vi "test_OpenClose (Multi Sessions) 2.vi"() -> ()   [LabVIEW 2020]
uses:
  <instrlib>/AIM GmbH/_AIM 664/AIM664LV.lvlib
  <instrlib>/AIM GmbH/_AIM 664/bsp/Fdx Create Session (Tx-Generic).vi
panel:
  in  "board 2":u32
  in  "port 2":u32
  in  "port":u32
  in  "board":u32
  out "executed":i32
  in  "Iterations":i32=1
  in  "idle before iterations mS":u32=1000
  out "error out 2":errorcluster caption="error out"
  out "error out":errorcluster
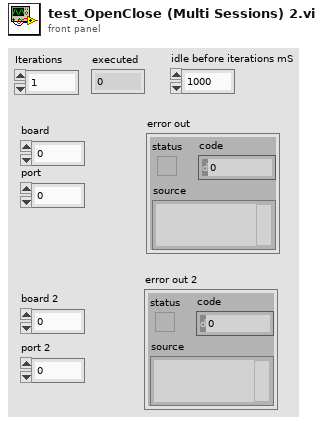
[diagram p1: front panel]
types:
  T1 = cluster{"ReceiveMode":u32, "DefaultPayloadMode":u32, "DefaultCronoMode":u32, "GlbMonBufferSizeIn":u32, "RerosDefaultOutputPortmap":u32}
  T2 = cluster{"ResourceID":u32, "ResourceType":u32, "ResourceInfo":string, "StructId":u32}
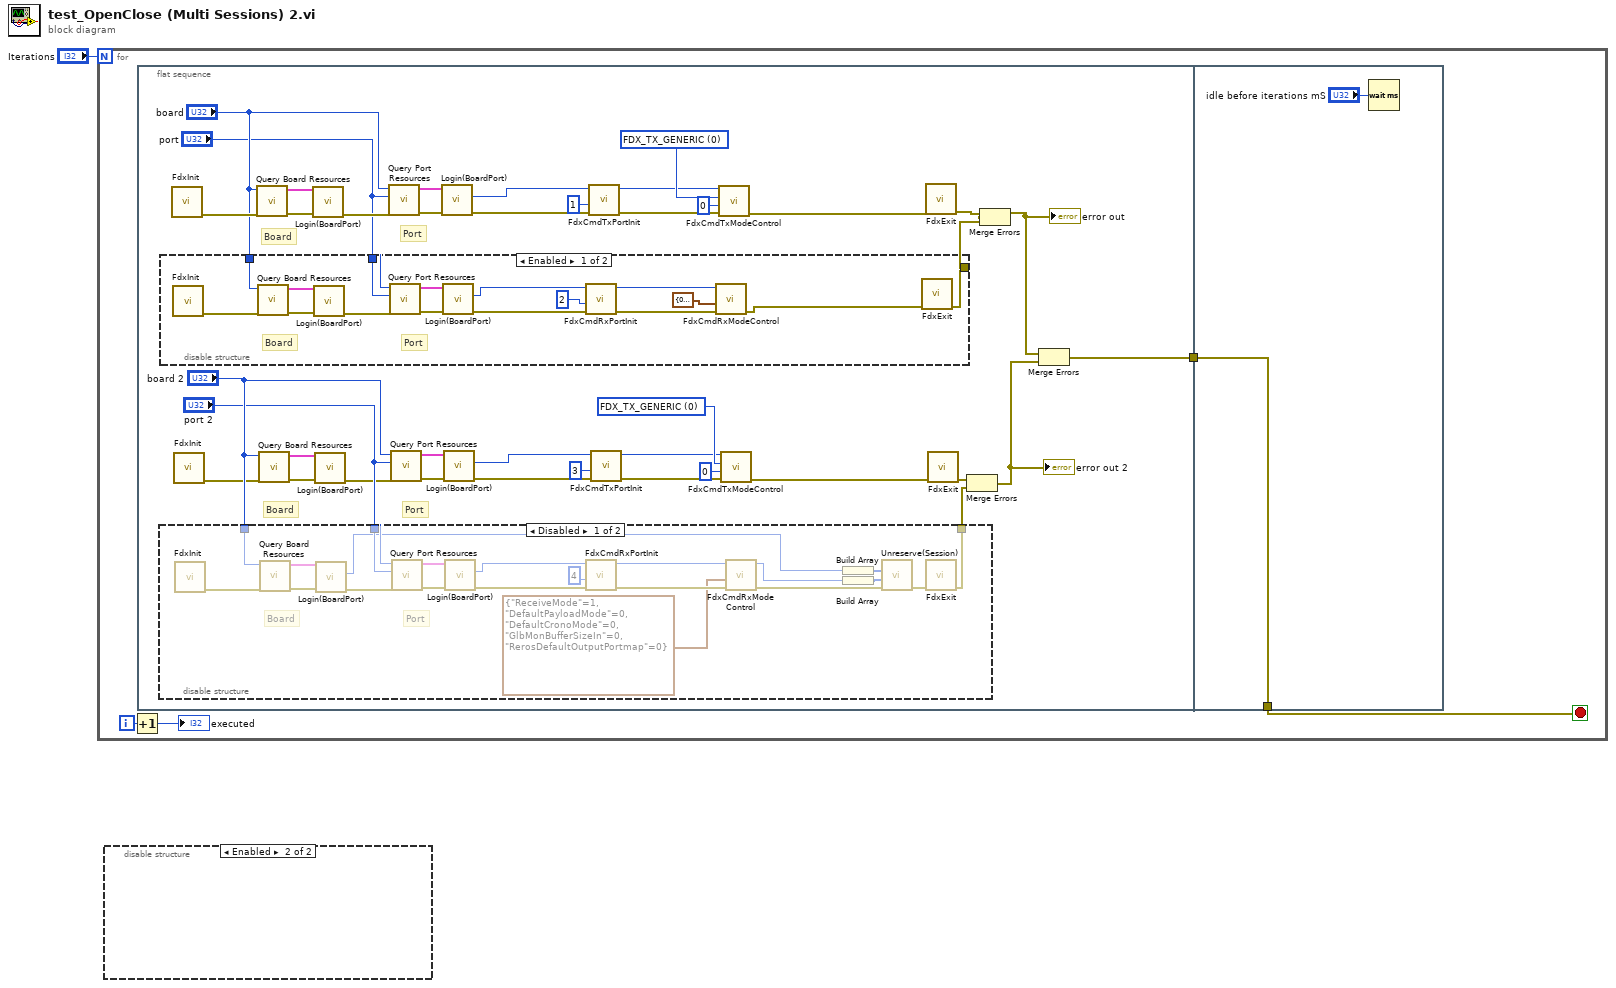
[diagram p0: block diagram]
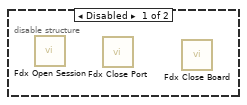
[diagram p4: hidden frame]
diagram:
  n1 = for {
    N: "Iterations" -> [_]
    i -> [w3]
    stop <- w5 stop-if-true
    n2 = Increment(x=w3) -> (x+1=→"executed":i32)
    n3 = flat-sequence {
      tunnel: [w44] -> w4
      tunnel: [w82] -> w5
      tunnel: w4 -> [w82]
      frame #0 {
        w28 = u32 0 items=["FDX_TX_GENERIC", "FDX_TX_REPLAY", "FDX_TX_INDIVIDUAL"] ("TransmitMode")
        w36 = u32 0 items=["FDX_TX_GENERIC", "FDX_TX_REPLAY", "FDX_TX_INDIVIDUAL"] ("TransmitMode")
        # "Port"
        # "Board"
        # "Port"
        # "Board"
        n4 = disable-structure shown="Disabled" {
          disable-tunnel: "board 2" -> [w75 _]
          disable-tunnel: "port 2" -> [w74 _]
          disable-tunnel: [w64 _] -> w22
          frame Disabled {
            # "Port"
            # "Board"
            n5 = call <instrlib>:"FdxInit.vi"() -> ("error out"=w81:errorcluster)  [unwired: 10 in, 1 out]
            n6 = call <instrlib>:"Query Board Resources.vi"("error in (no error)"=w81, "board"=w75) -> ("error out"=w80:errorcluster, "board resource"=w79:T2)  [unwired: 7 in, 1 out]
            n7 = call <instrlib>:"Login(BoardPort).vi"("error in (no error)"=w80, "resource in"=w79) -> ("error out"=w78:errorcluster, "Handle"=w70:u32)  [unwired: 7 in, 1 out]
            n8 = call <instrlib>:"Query Port Resources.vi"("error in (no error)"=w78, "port"=w74, "board"=w75) -> ("error out"=w77:errorcluster, "port resource"=w76:T2)  [unwired: 6 in, 1 out]
            n9 = call <instrlib>:"Login(BoardPort).vi"("error in (no error)"=w77, "resource in"=w76) -> ("error out"=w69:errorcluster, "Handle"=w62:u32)  [unwired: 7 in, 1 out]
            n10 = call <instrlib>:"FdxCmdRxPortInit.vi"("error in"=w69, "PortMap"=u32 4, "InstrumentHandle_port in"=w62) -> ("error out"=w68:errorcluster, "InstrumentHandle_port out"=w63:u32)  [unwired: 6 in, 1 out]
            n11 = call <instrlib>:"FdxCmdRxModeControl.vi"("error in"=w68, "RxModeControlIn"=T1 {"ReceiveMode"=1, "DefaultPayloadMode"=0, "DefaultCronoMode"=0, "GlbMonBufferSizeIn"=0, "RerosDefaultOutputPortmap"=0}, "InstrumentHandle_port in"=w63) -> ("error out"=w67:errorcluster, "InstrumentHandle_port out"=w66:u32)  [unwired: 6 in, 1 out]
            n12 = Build Array(w70) -> (w71:u32[])
            n13 = Build Array(w66) -> (w72:u32[])
            n14 = call <instrlib>:"Unreserve(Session).vi"("error in (no error)"=w67, "InstrumentHandle_port in"=w72, "InstrumentHandle_board in"=w71) -> ("error out"=w73:errorcluster)  [unwired: 8 in]
            n15 = call <instrlib>:"FdxExit.vi"("error in"=w73) -> ("error out"=w64:errorcluster)  [unwired: 10 in]
          }
          frame Enabled {
          }
        }
        n16 = disable-structure shown="Enabled" {
          disable-tunnel: [w52 _] -> w23
          disable-tunnel: "board" -> [w51 _]
          disable-tunnel: "port" -> [w50 _]
          frame Enabled {
            # "Port"
            # "Board"
            n17 = call <instrlib>:"FdxInit.vi"() -> ("error out"=w55:errorcluster)  [unwired: 10 in, 1 out]
            n18 = call <instrlib>:"Query Board Resources.vi"("error in (no error)"=w55, "board"=w51) -> ("error out"=w56:errorcluster, "board resource"=w57:T2)  [unwired: 7 in, 1 out]
            n19 = call <instrlib>:"Login(BoardPort).vi"("error in (no error)"=w56, "resource in"=w57) -> ("error out"=w58:errorcluster)  [unwired: 7 in, 2 out]
            n20 = call <instrlib>:"Query Port Resources.vi"("error in (no error)"=w58, "port"=w50, "board"=w51) -> ("error out"=w59:errorcluster, "port resource"=w60:T2)  [unwired: 6 in, 1 out]
            n21 = call <instrlib>:"Login(BoardPort).vi"("error in (no error)"=w59, "resource in"=w60) -> ("error out"=w54:errorcluster, "Handle"=w49:u32)  [unwired: 7 in, 1 out]
            n22 = call <instrlib>:"FdxCmdRxPortInit.vi"("error in"=w54, "PortMap"=u32 2, "InstrumentHandle_port in"=w49) -> ("error out"=w53:errorcluster, "InstrumentHandle_port out"=w47:u32)  [unwired: 6 in, 1 out]
            n23 = call <instrlib>:"FdxCmdRxModeControl.vi"("error in"=w53, "RxModeControlIn"=T1 {"ReceiveMode"=0, "DefaultPayloadMode"=0, "DefaultCronoMode"=0, "GlbMonBufferSizeIn"=0, "RerosDefaultOutputPortmap"=0}, "InstrumentHandle_port in"=w47) -> ("error out"=w46:errorcluster)  [unwired: 6 in, 2 out]
            n24 = call <instrlib>:"FdxExit.vi"("error in"=w46) -> ("error out"=w52:errorcluster)  [unwired: 10 in]
          }
          frame Disabled {
          }
        }
        n25 = call <instrlib>:"FdxInit.vi"() -> ("error out"=w43:errorcluster)  [unwired: 10 in, 1 out]
        n26 = call <instrlib>:"FdxInit.vi"() -> ("error out"=w7:errorcluster)  [unwired: 10 in, 1 out]
        n27 = call <instrlib>:"Query Board Resources.vi"("error in (no error)"=w43, "board"="board") -> ("error out"=w42:errorcluster, "board resource"=w41:T2)  [unwired: 7 in, 1 out]
        n28 = call <instrlib>:"Query Board Resources.vi"("error in (no error)"=w7, "board"="board 2") -> ("error out"=w8:errorcluster, "board resource"=w9:T2)  [unwired: 7 in, 1 out]
        n29 = call <instrlib>:"Login(BoardPort).vi"("error in (no error)"=w42, "resource in"=w41) -> ("error out"=w40:errorcluster)  [unwired: 7 in, 2 out]
        n30 = call <instrlib>:"Login(BoardPort).vi"("error in (no error)"=w8, "resource in"=w9) -> ("error out"=w10:errorcluster)  [unwired: 7 in, 2 out]
        n31 = call <instrlib>:"Query Port Resources.vi"("error in (no error)"=w40, "port"="port", "board"="board") -> ("error out"=w39:errorcluster, "port resource"=w38:T2)  [unwired: 6 in, 1 out]
        n32 = call <instrlib>:"Query Port Resources.vi"("error in (no error)"=w10, "port"="port 2", "board"="board 2") -> ("error out"=w11:errorcluster, "port resource"=w12:T2)  [unwired: 6 in, 1 out]
        n33 = call <instrlib>:"Login(BoardPort).vi"("error in (no error)"=w39, "resource in"=w38) -> ("error out"=w31:errorcluster, "Handle"=w30:u32)  [unwired: 7 in, 1 out]
        n34 = call <instrlib>:"Login(BoardPort).vi"("error in (no error)"=w11, "resource in"=w12) -> ("error out"=w17:errorcluster, "Handle"=w18:u32)  [unwired: 7 in, 1 out]
        n35 = call <instrlib>:"FdxCmdTxPortInit.vi"("error in"=w31, "PortMap"=u32 1, "InstrumentHandle_port"=w30) -> ("error out"=w33:errorcluster, "InstrumentHandle_port"=w35:u32)  [unwired: 6 in, 1 out]
        n36 = call <instrlib>:"FdxCmdTxPortInit.vi"("error in"=w17, "PortMap"=u32 3, "InstrumentHandle_port"=w18) -> ("error out"=w15:errorcluster, "InstrumentHandle_port"=w13:u32)  [unwired: 6 in, 1 out]
        n37 = call <instrlib>:"FdxCmdTxModeControl.vi"("error in"=w33, "RerosPortDelay"=u32 0, "TransmitMode"=w36, "InstrumentHandle_port"=w35) -> ("error out"=w32:errorcluster)  [unwired: 6 in, 1 out]
        n38 = call <instrlib>:"FdxCmdTxModeControl.vi"("error in"=w15, "RerosPortDelay"=u32 0, "TransmitMode"=w28, "InstrumentHandle_port"=w13) -> ("error out"=w16:errorcluster)  [unwired: 6 in, 1 out]
        n39 = call <instrlib>:"FdxExit.vi"("error in"=w32) -> ("error out"=w37:errorcluster)  [unwired: 10 in]
        n40 = call <instrlib>:"FdxExit.vi"("error in"=w16) -> ("error out"=w6:errorcluster)  [unwired: 10 in]
        n41 = Merge Errors(w6, w22) -> (w26:errorcluster)
        "error out 2" <- w26
        n42 = Merge Errors(w37, w23) -> (w27:errorcluster)
        "error out" <- w27
        n43 = Merge Errors(w27, w26) -> (w44:errorcluster)
      }
      frame #1 {
        n44 = Wait (ms)(milliseconds to wait="idle before iterations mS") -> ()  [unwired: 1 out]
      }
    }
  }
  n45 = disable-structure shown="Enabled" {
    frame Disabled {
      n46 = call-poly <instrlib>:"Fdx Open Session.vi"() -> ()  [unwired: 6 in, 6 out]
      n47 = call <instrlib>:"Fdx Close Port.vi"() -> ()  [unwired: 10 in, 2 out]
      n48 = call <instrlib>:"Fdx Close Board.vi"() -> ()  [unwired: 11 in, 1 out]
    }
    frame Enabled {
    }
  }
